vi "Tektronix TDS 200 1000 2000 Series Acquire Measurement.vi"() -> ()   [LabVIEW 2012]
doc: "This example shows how to configure two channels and acquire measurement from multiple channels.\n\n<B>Notes:</B>\nAvailable on TBS1000B-EDU, TBS1000B and TDS2000C series only."
uses:
  <instrlib>/Tektronix TDS 200 1000 2000 Series/Tektronix TDS 200 1000 2000 Series.lvlib
panel:
  out "Units":string
  out "Measurement":dbl
  in  "Measurement Type (0: Phase)":u16(ring) items=["Phase", "Delay", "DelayRR", "DelayRF", "DelayFR", "DelayFF"]
  in  "Channel B (1: Channel 2)":u16(ring)=1 items=["Channel 1", "Channel 2", "Channel 3", "Channel 4"]
  in  "Channel A (0: Channel 1)":u16(ring) items=["Channel 1", "Channel 2", "Channel 3", "Channel 4"]
  in  "Serial Configuration":T1={"Baud Rate"=9600, "Parity"=0, "Stop Bits"=10, "Flow Control"=2} {"Flow Control" items=["None", "XON/XOFF", "RTS/CTS", "XON/XOFF & RTS/CTS", "DTR/DSR", "XON/XOFF & DTR/DSR"]; "Stop Bits" items=["1.0"=10, "1.5"=15, "2.0"=20]; "Parity" items=["None", "Odd", "Even", "Mark", "Space"]; "Baud Rate" items=["300"=300, "600"=600, "1200"=1200, "2400"=2400, "4800"=4800, "9600"=9600, "19200"=19200]}
  in  "Probe Attenuation B (1.0)":dbl=1.0
  in  "Vertical Coupling B (1: DC)":u16(ring)=1 items=["AC", "DC", "Ground"]
  in  "Probe Attenuation A (10.0)":dbl=10.0
  in  "Vertical Coupling A (1: DC)":u16(ring)=1 items=["AC", "DC", "Ground"]
  in  "VISA resource name":refnum<visa-resource-name>
  # "(C) 2014 National Instruments.  ALL RIGHTS RESERVED."
  # "Channel A"
  # "Channel B"
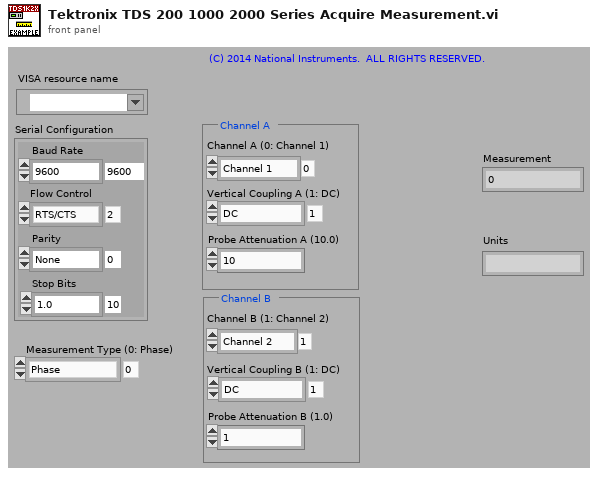
[diagram p1: front panel]
types:
  T1 = cluster{"Baud Rate":u32, "Parity":u16, "Stop Bits":u16, "Flow Control":u16}
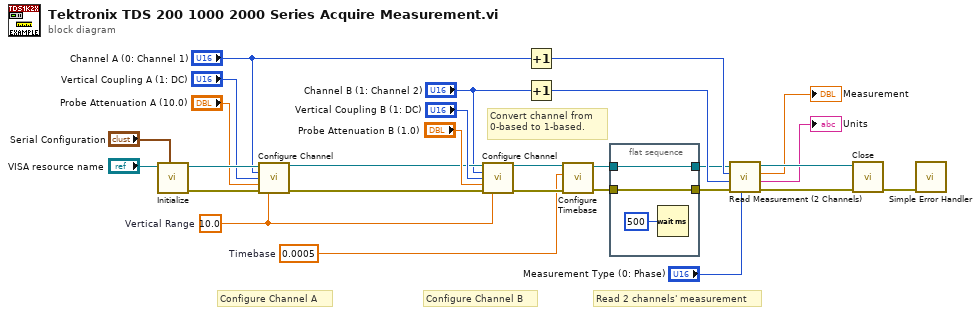
[diagram p0: block diagram]
diagram:
  w18 = 10.0  # Vertical Range
  w17 = 0.0005  # Timebase
  # "Read 2 channels' measurement"
  # "Convert channel from\n0-based to 1-based."
  # "Configure Channel B"
  # "Configure Channel A"
  n1 = call <instrlib>:"Initialize.vi"("Serial Configuration"="Serial Configuration", "VISA resource name"="VISA resource name") -> ("error out"=w25:errorcluster, "VISA resource name out"=w26:refnum<visa-resource-name>)  [unwired: 3 in, 5 out]
  n2 = call <instrlib>:"Configure Channel.vi"("VISA resource name"=w26, "Channel (0: Channel 1)"="Channel A (0: Channel 1)", "Vertical Coupling (1: DC)"="Vertical Coupling A (1: DC)", "Probe Attenuation (10: 10X)"="Probe Attenuation A (10.0)", "error in (no error)"=w25, "Vertical Range (10.0 V/div)"=w18) -> ("VISA resource name out"=w15:refnum<visa-resource-name>, "error out"=w14:errorcluster)  [unwired: 3 in, 5 out]
  n3 = call <instrlib>:"Configure Channel.vi"("VISA resource name"=w15, "Channel (0: Channel 1)"="Channel B (1: Channel 2)", "Vertical Coupling (1: DC)"="Vertical Coupling B (1: DC)", "Probe Attenuation (10: 10X)"="Probe Attenuation B (1.0)", "error in (no error)"=w14, "Vertical Range (10.0 V/div)"=w18) -> ("VISA resource name out"=w24:refnum<visa-resource-name>, "error out"=w23:errorcluster)  [unwired: 3 in, 5 out]
  n4 = Increment(x="Channel A (0: Channel 1)") -> (x+1=w7:u16)
  n5 = Increment(x="Channel B (1: Channel 2)") -> (x+1=w5:u16)
  n6 = call <instrlib>:"Configure Timebase.vi"("error in (no error)"=w23, "Timebase (0.0005 s)"=w17, "VISA resource name"=w24) -> ("error out"=w1:errorcluster, "VISA resource name out"=w4:refnum<visa-resource-name>)  [unwired: 1 in, 6 out]
  n7 = flat-sequence {
    tunnel: w4 -> [w31]
    tunnel: [w31] -> w3
    tunnel: w1 -> [w30]
    tunnel: [w30] -> w2
    frame #0 {
      n8 = Wait (ms)(milliseconds to wait=u32 500) -> ()  [unwired: 1 out]
    }
  }
  n9 = call <instrlib>:"Read Measurement (2 Channels).vi"("Measurement Type (0: Phase)"="Measurement Type (0: Phase)", "error in (no error)"=w2, "Channel 2 (2: Channel 2)"=w5, "Channel 1 (1: Channel 1)"=w7, "VISA resource name"=w3) -> ("error out"=w11:errorcluster, "Units"=→"Units":string, "Measurement"=→"Measurement":dbl, "VISA resource name out"=w12:refnum<visa-resource-name>)  [unwired: 3 out]
  n10 = call <instrlib>:"Close.vi"("error in (no error)"=w11, "VISA resource name"=w12) -> ("error out"=w27:errorcluster)  [unwired: 9 out]
  n11 = call <vilib>:"Simple Error Handler.vi"("error in (no error)"=w27) -> ()  [unwired: 1 in, 8 out]
